vi "Reward FB (SubVI).vi"(9 "# each state":i32[](array[numeric])=[1000, 100], 10 "Action":i32, 11 "State":i32) -> (3 "Reward":dbl)   [LabVIEW 2013]
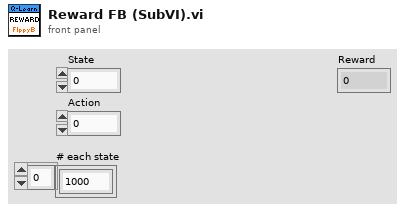
[diagram p1: front panel]
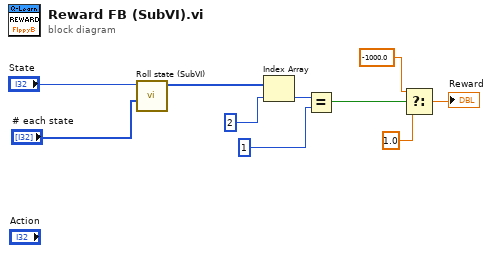
[diagram p0: block diagram]
diagram:
  n1 = call "Roll state (SubVI).vi"("# each state"="# each state", "Unrolled state"="State") -> ("State array"=w10:i32[])  [unwired: 9 in]
  n2 = Index Array(array=w10, index=2) -> (element=w8:i32)
  n3 = Equal?(x=w8, y=1 ("x")) -> (x = y?=w7:bool)
  n4 = Select(t=-1000.0, s=w7, f=1.0) -> (s? t:f=→"Reward":dbl)
